vi "PASS OR FAIL.vi"() -> ()   [LabVIEW 2018]
panel:
  out "RESULT":bool
  in  "MARKS":i32
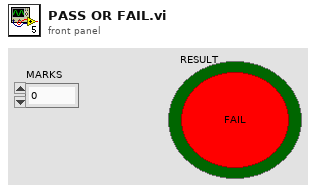
[diagram p1: front panel]
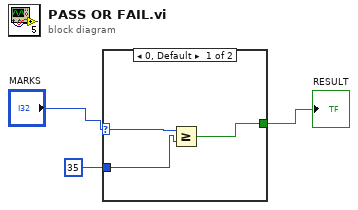
[diagram p0: block diagram]
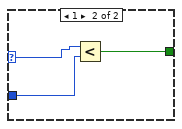
[diagram p2: hidden frame]
diagram:
  n1 = case shown="0, Default" "MARKS" {
    selector: "MARKS" -> [w6 w7]
    tunnel: [w4 w9] -> w2
    tunnel: 35 ("y") -> [w5 w8]
    frame 0, Default {
      n2 = Greater Or Equal?(x=w6, y=w5) -> (x >= y?=w4:bool)
    }
    frame 1 {
      n3 = Less?(x=w7, y=w8) -> (x < y?=w9:bool)
    }
  }
  "RESULT" <- w2
